vi "Rx Int Close Event.vi"(10 "hEvt":u32, 11 "devId":i32) -> (2 "hEvt out":u32, 3 "function return":i32)   [LabVIEW 2013, in "CHR34XXX.lvlib"]
doc: "DLL BOOL __stdcall CHR34XXX_RxInt_CloseEvent(IN int devId,IN HANDLE hEvt);"
uses:
  CHR34XXX.lvlib
  CHR34XXX.dll
panel:
  out "devId out":i32
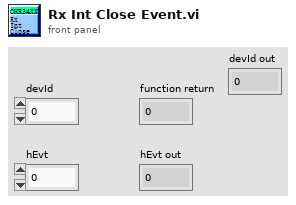
[diagram p1: front panel]
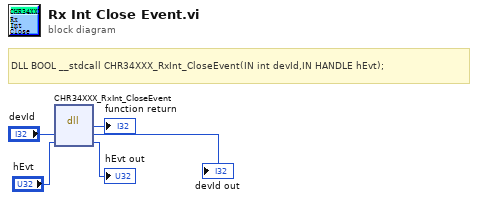
[diagram p0: block diagram]
diagram:
  # "DLL BOOL __stdcall CHR34XXX_RxInt_CloseEvent(IN int devId,IN HANDLE hEvt);"
  n1 = dll-call lib="C:/Users/Administrator/Desktop/CHR34XXX_lv/lv_lib/CHR34XXX.*" fn="CHR34XXX_RxInt_CloseEvent"("devId"="devId", "hEvt"="hEvt") -> (→"function return":i32, "devId"=→"devId out":i32, "hEvt"=→"hEvt out":u32)  [unwired: 3 in, 2 out]
